vi "Create Data Server.vi"(5 "data server options":T1={"Enable Data Server"=FALSE, "Period"=100} {"Period" format="%d ms"}, 7 "Framework Configuration":refnum<class "Framework Configuration.lvclass">, 8 "error in (no error)":errorcluster, 10 "Plugins":refnum<class "Plugin.lvclass">[](array[class]), 11 "Framework in":refnum<class "Framework.lvclass">) -> (0 "error out":errorcluster, 2 "Data Server Thread":refnum<class "Data Server Thread.lvclass">, 3 "Framework out":refnum<class "Framework.lvclass">)   [LabVIEW 2017, in "DSF Core.lvlib" / "Framework.lvclass"]
uses:
  Framework.lvclass
  Plugin/Plugin.lvclass
  Thread/Data Server/Data Server Thread.lvclass
  Data Server Options.ctl
  Configuration/Framework/Framework Configuration.lvclass
  Thread/Data Server/Framework.ctl
  Buffers/Buffers.lvclass
  Status/Status Pointer.lvclass
  Thread/Data Server/Plugin.ctl
  Thread/Data Server/Group.ctl
  Transfer/Transfer.lvclass
  Framework.lvclass/Framework.ctl
  Transfer Group/Transfer Group.lvclass
  Framework Status/Framework Status.lvclass
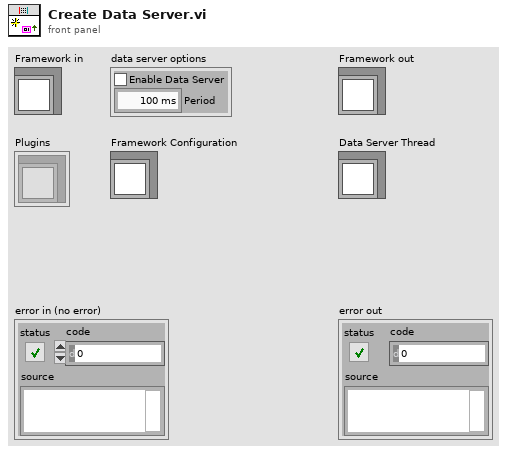
[diagram p1: front panel]
types:
  T1 = typedef "DSF Core.lvlib/Framework.lvclass/Data Server Options.ctl" = cluster{"Enable Data Server":bool, "Period":u32}
  T2 = typedef "DSF Core.lvlib/Data Server Thread.lvclass/Framework.ctl" = cluster{"Framework Buffers":refnum<class "Buffers.lvclass">, "Framework Status":refnum<class "Status Pointer.lvclass">, "Plugins":T3[]}
  T3 = typedef "DSF Core.lvlib/Data Server Thread.lvclass/Plugin.ctl" = cluster{"Plugin Buffers":refnum<class "Buffers.lvclass">, "Plugin Status":refnum<class "Status Pointer.lvclass">, "Groups":T4[]}
  T4 = typedef "DSF Core.lvlib/Data Server Thread.lvclass/Group.ctl" = cluster{"Group Buffers":refnum<class "Buffers.lvclass">, "Group Status":refnum<class "Status Pointer.lvclass">, "Transfers":refnum<class "Transfer.lvclass">[]}
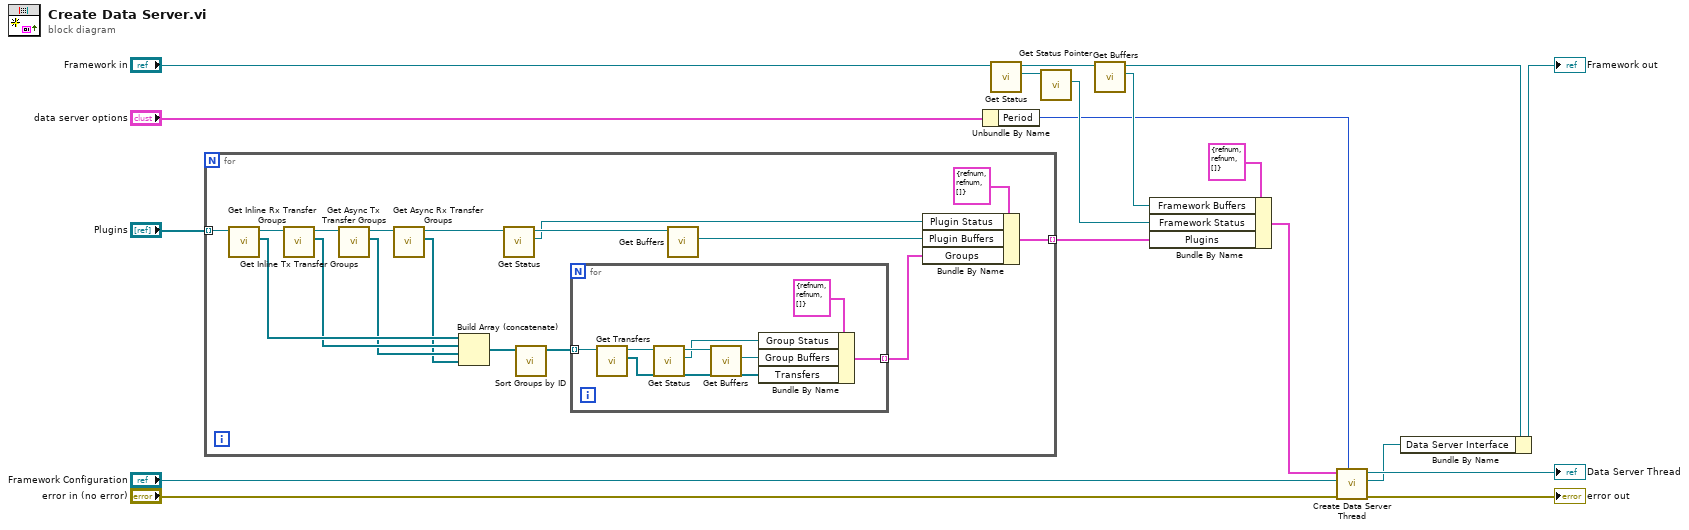
[diagram p0: block diagram]
diagram:
  n1 = for {
    tunnel: "Plugins" -> [w32] mode=indexing
    tunnel: [w34] -> w9 mode=indexing
    n2 = call "Get Inline Rx Transfer Groups.vi"("Plugin in"=w32) -> ("Inline Rx Transfer Groups"=w28:refnum<class "Transfer Group.lvclass">[], "Plugin out"=w31:refnum<class "Plugin.lvclass">)  [unwired: 9 in]
    n3 = call "Get Inline Tx Transfer Groups.vi"("Plugin in"=w31) -> ("Inline Tx Transfer Groups"=w27:refnum<class "Transfer Group.lvclass">[], "Plugin out"=w30:refnum<class "Plugin.lvclass">)  [unwired: 9 in]
    n4 = call "Get Async Tx Transfer Groups.vi"("Plugin in"=w30) -> ("Async Tx Transfer Groups"=w26:refnum<class "Transfer Group.lvclass">[], "Plugin out"=w29:refnum<class "Plugin.lvclass">)  [unwired: 9 in]
    n5 = call "Get Async Rx Transfer Groups.vi"("Plugin in"=w29) -> ("Async Rx Transfer Groups"=w24:refnum<class "Transfer Group.lvclass">[], "Plugin out"=w21:refnum<class "Plugin.lvclass">)  [unwired: 9 in]
    n6 = Build Array (concatenate)(w28, w27, w26, w24) -> (w25:refnum<class "Transfer Group.lvclass">[])
    n7 = call "Get Status.vi"("Plugin in"=w21) -> ("status pointer"=w19:refnum<class "Status Pointer.lvclass">, "Plugin out"=w20:refnum<class "Plugin.lvclass">)  [unwired: 9 in]
    n8 = call "Sort Groups by ID.vi"("Transfers Groups in"=w25) -> ("ID-sorted Transfers Groups out"=w23:refnum<class "Transfer Group.lvclass">[])  [unwired: 9 in, 1 out]
    n9 = for {
      tunnel: w23 -> [w40] mode=indexing
      tunnel: [w41] -> w22 mode=indexing
      n10 = call "Get Transfers.vi"("Transfer Group in"=w40) -> ("Transfers"=w39:refnum<class "Transfer.lvclass">[], "Transfer Group out"=w38:refnum<class "Transfer Group.lvclass">)  [unwired: 9 in]
      n11 = call "Get Status.vi"("Transfer Group in"=w38) -> ("status pointer"=w36:refnum<class "Status Pointer.lvclass">, "Transfer Group out"=w37:refnum<class "Transfer Group.lvclass">)  [unwired: 9 in]
      n12 = call "Get Buffers.vi"("Transfer Group in"=w37) -> ("Buffers"=w42:refnum<class "Buffers.lvclass">)  [unwired: 9 in, 1 out]
      n13 = Bundle By Name(cluster=T4 {"Group Buffers"=refnum, "Group Status"=refnum, "Transfers"=[]} ("Group"), "Group Status"=w36, "Group Buffers"=w42, "Transfers"=w39) -> (w41:T4)
    }
    n14 = call "Get Buffers.vi"("Plugin in"=w20) -> ("Buffers"=w33:refnum<class "Buffers.lvclass">)  [unwired: 9 in, 1 out]
    n15 = Bundle By Name(cluster=T3 {"Plugin Buffers"=refnum, "Plugin Status"=refnum, "Groups"=[]} ("Plugin"), "Plugin Status"=w19, "Plugin Buffers"=w33, "Groups"=w22) -> (w34:T3)
  }
  n16 = Unbundle By Name("data server options") -> ("Period"=w1:u32)
  n17 = call "Get Status.vi"("Framework in"="Framework in") -> ("Status"=w6:refnum<class "Framework Status.lvclass">, "Framework out"=w4:refnum<class "Framework.lvclass">)  [unwired: 9 in]
  n18 = call "Get Status Pointer.vi"("Framework Status in"=w6) -> ("status pointer"=w5:refnum<class "Status Pointer.lvclass">)  [unwired: 8 in, 2 out]
  n19 = call "Get Buffers.vi"("Framework in"=w4) -> ("Buffers"=w2:refnum<class "Buffers.lvclass">, "Framework out"=w3:refnum<class "Framework.lvclass">)  [unwired: 9 in]
  n20 = Bundle By Name(cluster=T2 {"Framework Buffers"=refnum, "Framework Status"=refnum, "Plugins"=[]} ("Buffers"), "Framework Buffers"=w2, "Framework Status"=w5, "Plugins"=w9) -> (w8:T2)
  n21 = call "Create Data Server Thread.vi"("period (100 ms)"=w1, "error in (no error)"="error in (no error)", "Framework Configuration"="Framework Configuration", "Buffers"=w8) -> ("error out"=→"error out":errorcluster, "Interface"=w13:refnum<class "Plugin Interface.lvclass">, "Data Server Thread out"=→"Data Server Thread":refnum<class "Data Server Thread.lvclass">)  [unwired: 5 in]
  n22 = Bundle By Name(cluster=w3, "Data Server Interface"=w13) -> (→"Framework out":refnum<class "Framework.lvclass">)
